vi "获取设备属性.vi"() -> ()   [LabVIEW 2013]
panel:
  out "AI最大采样频率":dbl
  out "AI通道数":u32
  out "产品序列号":u32
  out "产品名称":string
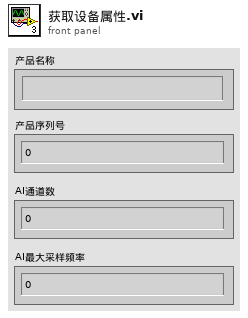
[diagram p1: front panel]
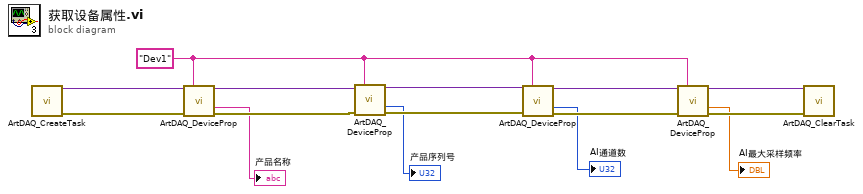
[diagram p0: block diagram]
diagram:
  w5 = "Dev1" ("设备名称")
  n1 = call <userlib>:"ArtDAQ_CreateTask.vi"() -> ("任务句柄"=w15:variant, "错误输出"=w14:errorcluster)  [unwired: 14 in]
  n2 = call-poly <userlib>:"ArtDAQ_DeviceProp.vi"("任务句柄"=w15, "设备名称"=w5, "错误输入"=w14) -> ("任务句柄"=w13:variant, "产品名称"=→"产品名称":string, "错误输出"=w12:errorcluster)  [unwired: 10 in]
  n3 = call-poly <userlib>:"ArtDAQ_DeviceProp.vi"("任务句柄"=w13, "设备名称"=w5, "错误输入"=w12) -> ("任务句柄"=w11:variant, "产品序列号"=→"产品序列号":u32, "错误输出"=w10:errorcluster)  [unwired: 10 in]
  n4 = call-poly <userlib>:"ArtDAQ_DeviceProp.vi"("任务句柄"=w11, "设备名称"=w5, "错误输入"=w10) -> ("任务句柄"=w9:variant, "AI通道数"=→"AI通道数":u32, "错误输出"=w8:errorcluster)  [unwired: 10 in]
  n5 = call-poly <userlib>:"ArtDAQ_DeviceProp.vi"("任务句柄"=w9, "设备名称"=w5, "错误输入"=w8) -> ("任务句柄"=w7:variant, "AI采样率"=→"AI最大采样频率":dbl, "错误输出"=w6:errorcluster)  [unwired: 10 in]
  n6 = call <userlib>:"ArtDAQ_ClearTask.vi"("任务句柄"=w7, "错误输入"=w6) -> ()  [unwired: 13 in, 1 out]
